vi "Get Waveform Sweep Status.vi"(8 "error in (no error)":errorcluster, 10 "index":i32, 11 "Waveforms in":waveform(dbl)[](array[waveform])) -> (0 "error out":errorcluster, 2 "sweep status":T1, 3 "Waveforms out":waveform(dbl)[](array[waveform]))   [LabVIEW 2019, in "Waveform.Attributes.lvlib"]
uses:
  Waveform.Attributes.lvlib
  Generator/typedefs/Generator.Sweep Status--enum.ctl
  Generator/Generator.lvclass
  <vilib>/Waveform/WDTOps.llb/WDT Number of Waveform Samples DBL.vi
panel:
  out "number of samples":i32
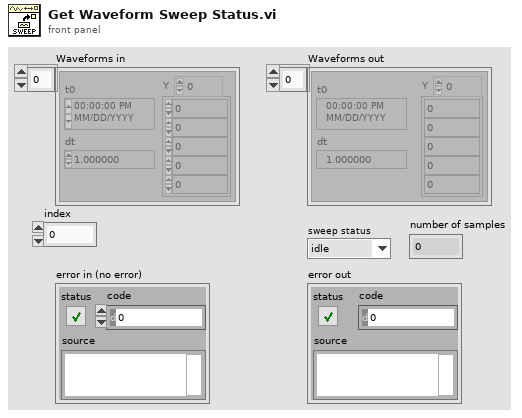
[diagram p1: front panel]
types:
  T1 = typedef "Generator.lvclass/Generator.Sweep Status--enum.ctl" = enum16{"idle", "initializing", "waiting", "sweeping", "stopping"}
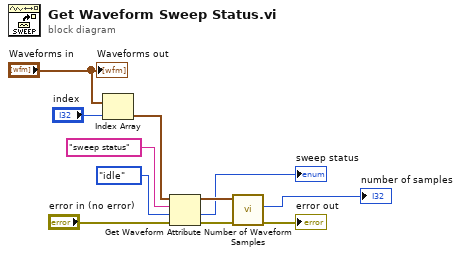
[diagram p0: block diagram]
diagram:
  n1 = Index Array(array="Waveforms in", index="index") -> (element=w10:waveform(dbl))
  n2 = Get Waveform Attribute(4:"error in (no error)", 5:Generator.Sweep_Status--enum."idle" ("sweep status"), 6:"sweep status" ("name"), 7:w10) -> (0:w4:errorcluster, 1:→"sweep status":T1, 3:w5:waveform(dbl))  [unwired: 1 out]
  n3 = call-poly <vilib>:"Number of Waveform Samples.vi"("error in (no error)"=w4, "waveform in"=w5) -> ("error out"=→"error out":errorcluster, "number of samples"=→"number of samples":i32)  [unwired: 7 in, 1 out]
  "Waveforms out" <- "Waveforms in"
